vi "dew-point.vi"(1 "H%":dbl, 2 "T°":dbl) -> (0 "T° pdr":dbl)   [LabVIEW 2010]
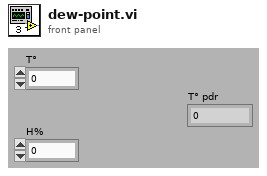
[diagram p1: front panel]
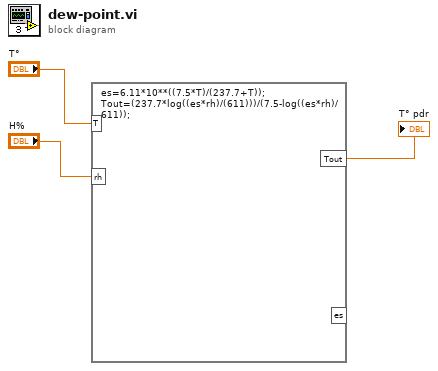
[diagram p0: block diagram]
diagram:
  n1 = formula code="es=6.11*10**((7.5*T)/(237.7+T));\nTout=(237.7*log((es*rh)/(611)))/(7.5-log((es*rh)/611));"("T"="T°", "rh"="H%") -> ("Tout"=→"T° pdr":dbl)  [unwired: 1 out]
